vi "Read Sync Box Setup.vi"(8 "error in (no error)":errorcluster, 11 "Interface in":refnum<class "Interface.lvclass">) -> (0 "error out":errorcluster, 3 "Interface out":refnum<class "Interface.lvclass">)   [LabVIEW 2018, in "Interface.lvclass"]
uses:
  Interface.lvclass
  Interface.lvclass/Interface.ctl
panel:
  out "Address":string
  out "Remote Port":u32
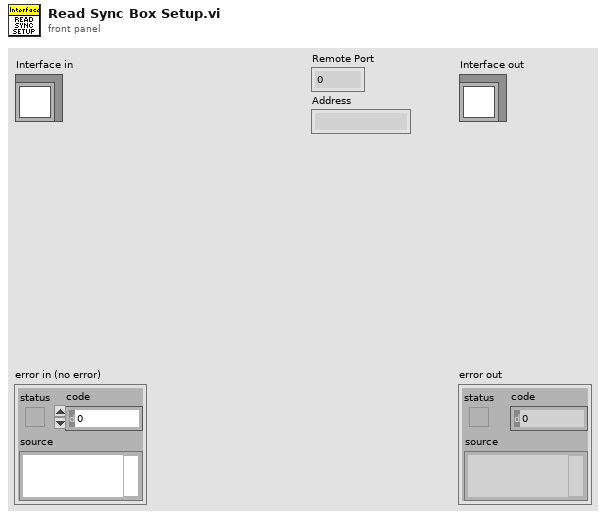
[diagram p1: front panel]
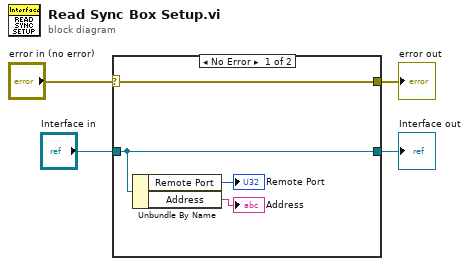
[diagram p0: block diagram]
diagram:
  n1 = case shown="No Error" "error in (no error)" {
    selector: "error in (no error)" -> [w8 w10]
    tunnel: [w8 w10] -> w3
    tunnel: [w7 w9] -> w1
    tunnel: "Interface in" -> [w7 w9]
    frame No Error {
      n2 = Unbundle By Name(w7) -> ("Remote Port"=→"Remote Port":u32, "Address"=→"Address":string)
    }
    frame Error {
    }
  }
  "error out" <- w3
  "Interface out" <- w1
